vi "Stop Control.vi"(1 "Mode (Read)":T1) -> (0 "Stop?":bool)   [LabVIEW 2023]
uses:
  MLA Stop Mode.ctl
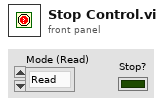
[diagram p1: front panel]
types:
  T1 = typedef "MLA Stop Mode.ctl" = enum16{"Read", "Set", "Reset"}
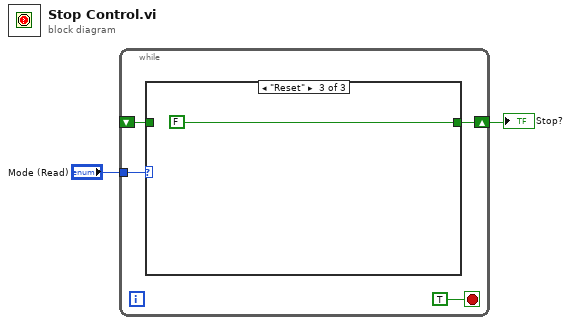
[diagram p0: block diagram]
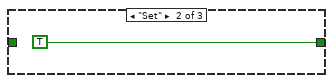
[diagram p3: hidden frame]
diagram:
  n1 = while {
    tunnel: "Mode (Read)" -> [w5]
    shift-right: [w4] -> w1
    shift-left: _ -> [w3]
    stop <- TRUE stop-if-true
    n2 = case shown="\"Reset\"" w5 {
      tunnel: [w7 TRUE FALSE] -> w4
      tunnel: w3 -> [w7 _ _]
      frame "Read" {
      }
      frame "Set" {
      }
      frame "Reset" {
      }
    }
  }
  "Stop?" <- w1
